vi "CheckCreateFile.vi"(8 "Error In":errorcluster, 10 "Folder":string, 11 "Image Name":string) -> (0 "Error Out":errorcluster, 3 "File Path":path)   [LabVIEW 2013]
doc: "VI Checks for a folder in the application\ndirectory. If it doesn't existe, the VI\ncreates the folder and returns the path of the\nimage that is being saved there. \n\nAlso checks to see if image already exists. If so, increments\nthe last number character before .jpg and saves the new image\nin the directory above."
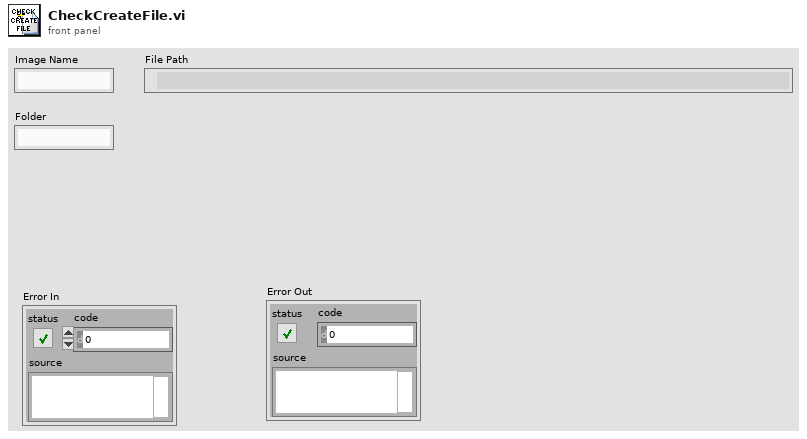
[diagram p1: front panel]
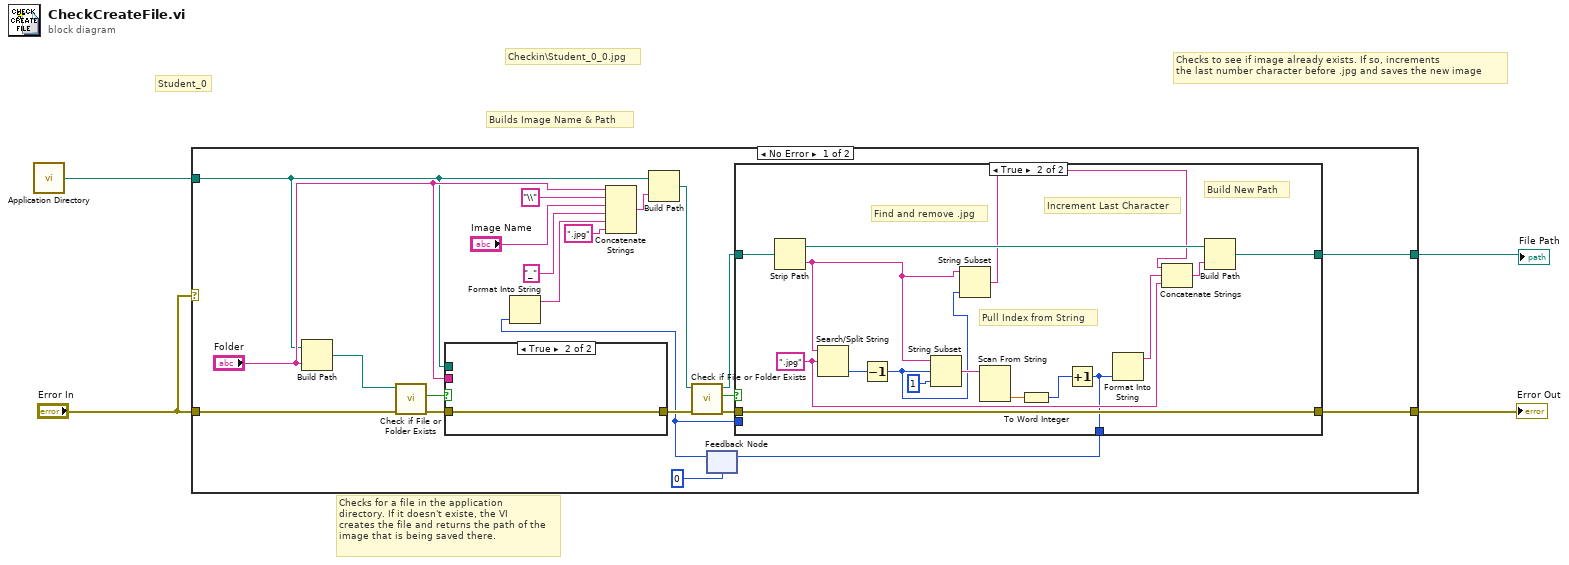
[diagram p0: block diagram]
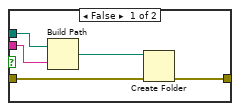
[diagram p3: hidden frame]
diagram:
  # "Checkin\\Student_0_0.jpg"
  # "Student_0"
  # "Builds Image Name & Path"
  # "Checks to see if image already exists. If so, increments\nthe last number character before .jpg and saves the new image"
  # "Checks for a file in the application\ndirectory. If it doesn't existe, the VI\ncreates the file and returns the path of the\nimage that is being saved there."
  n1 = call <vilib>:"Application Directory.vi"() -> ("Application Directory"=w1:path)
  n2 = case shown="No Error" "Error In" {
    tunnel: "Error In" -> [w12 w53]
    tunnel: [w11 w53] -> w4
    tunnel: [w9 w52] -> w2
    tunnel: w1 -> [w8 w52]
    frame No Error {
      n3 = Build Path(base path=w8, name or relative path="Folder") -> (appended path=w25:path)
      n4 = call <vilib>:"Check if File or Folder Exists.vi"("error in (no error)"=w12, "path"=w25) -> ("error out"=w26:errorcluster, "file or folder exists?"=w24:bool)  [unwired: 7 in, 1 out]
      n5 = case shown="True" w24 {
        tunnel: w8 -> [w50 _]
        tunnel: "Folder" -> [w48 _]
        tunnel: [w47 w51] -> w13
        tunnel: w26 -> [w46 w51]
        frame False {
          n6 = Build Path(base path=w50, name or relative path=w48) -> (appended path=w49:path)
          n7 = Create Folder(path (use dialog)=w49, error in=w46) -> (error out=w47:errorcluster)  [unwired: 1 in, 2 out]
        }
        frame True {
        }
      }
      n8 = feedback #1(0) -> (w5:i32)
      n9 = Format Into String(w5) -> (resulting string=w17:string)  [unwired: 3 in, 1 out]
      n10 = Concatenate Strings("Folder", "\\" ("string"), "Image Name", "_" ("string"), w17, ".jpg" ("string")) -> (w21:string)
      n11 = Build Path(base path=w8, name or relative path=w21) -> (appended path=w16:path)
      n12 = call <vilib>:"Check if File or Folder Exists.vi"("error in (no error)"=w13, "path"=w16) -> ("error out"=w10:errorcluster, "file or folder exists?"=w15:bool, "dup path"=w14:path)  [unwired: 7 in]
      n13 = case shown="True" w15 {
        tunnel: w14 -> [w29 w45]
        tunnel: [w29 w36] -> w9
        tunnel: [w28 w34] -> w11
        tunnel: w10 -> [w28 w34]
        tunnel: [w27 w30] -> w7
        tunnel: w5 -> [w27 _]
        frame False {
        }
        frame True {
          w38 = ".jpg" ("search string/char (-)")
          # "Build New Path"
          # "Increment Last Character"
          # "Find and remove .jpg"
          # "Pull Index from String"
          n14 = Strip Path(path=w45) -> (stripped path=w39:path, name=w33:string)
          n15 = Search/Split String(string=w33, search string/char (-)=w38) -> (offset of match=w43:i32)  [unwired: 1 in, 2 out]
          n16 = Decrement(x=w43) -> (x-1=w32:i32)
          n17 = String Subset(string=w33, offset (0)=w32, length (rest)=1 ("length (rest)")) -> (substring=w41:string)
          n18 = String Subset(string=w33, length (rest)=w32) -> (substring=w31:string)  [unwired: 1 in]
          n19 = Scan From String(input string=w41) -> (output 1=w42:dbl)  [unwired: 4 in, 3 out]
          n20 = To Word Integer(number=w42) -> (16bit integer=w35:i16)
          n21 = Increment(x=w35) -> (x+1=w30:i16)
          n22 = Format Into String(w30) -> (resulting string=w40:string)  [unwired: 3 in, 1 out]
          n23 = Concatenate Strings(w31, w40, w38) -> (w37:string)
          n24 = Build Path(base path=w39, name or relative path=w37) -> (appended path=w36:path)
        }
      }
      n25 = feedback-in #1(w7) -> ()
    }
    frame Error {
    }
  }
  "Error Out" <- w4
  "File Path" <- w2
